vi "main.vi"() -> ()   [LabVIEW 2011]
doc: "Use this template to build a producer/consumer design pattern. Use this template when you need to execute a process, such as data analysis, when a data source, such as a triggered acquisition, produces data at an uneven rate and you need to execute the process when the data becomes available."
uses:
  <vilib>/httpClient/POSTBuffer.vi
  <vilib>/httpClient/LabVIEWHTTPClient.lvlib
  Labview-JSON/src/JSON.lvlib
  <vilib>/addons/internet/NI_InternetTK_FTP_VIs.lvlib
panel:
  in  "host":string
  in  "ftpPassword":string
  in  "ftpUsername":string
  out "# elements":i32=1
  out "Size queue flushed":i32=1
  out "Queue size [bytes]":i32=44
  in  "Queue size limit [Kbytes]":i32=10
  in  "url":string="localhost:3001/datas"
  in  "password":string
  in  "username":string
  in  "stop":bool
  out "data queue too large":T1={"acc1"=0.11785432029080489, "vel1"=0.881508362393591, "f1"=0.32413347839367, "timestamp"=3413457307.4501805, "system"="system01"}
  out "data queue":T1={"acc1"=0.11785432029080489, "vel1"=0.881508362393591, "f1"=0.32413347839367, "timestamp"=3413457307.4501805, "system"="system01"}
  # "HTTP Config"
  # "FTP Config"
  # "Queue"
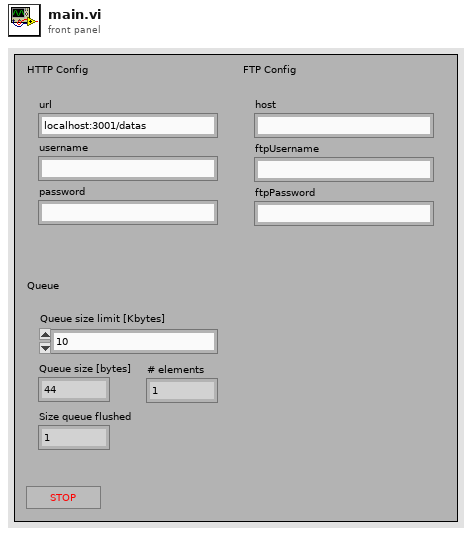
[diagram p1: front panel]
types:
  T1 = cluster{"acc1":dbl, "vel1":dbl, "f1":dbl, "timestamp":dbl, "system":string}
  T2 = cluster{"host":string, "ftpUsername":string, "ftpPassword":string, "ftpRemotePath":string}
  T3 = typedef "LabVIEWHTTPClient.lvlib/ClientHandle.ctl" = refnum<k1>
  T4 = enum16{"open", "replace", "create", "open or create", "replace or create", "replace or create with confirmation"}
  T5 = cluster{"acc1":dbl, "vel1":dbl, "f1":dbl, "timestamp":dbl, "system":string}[]
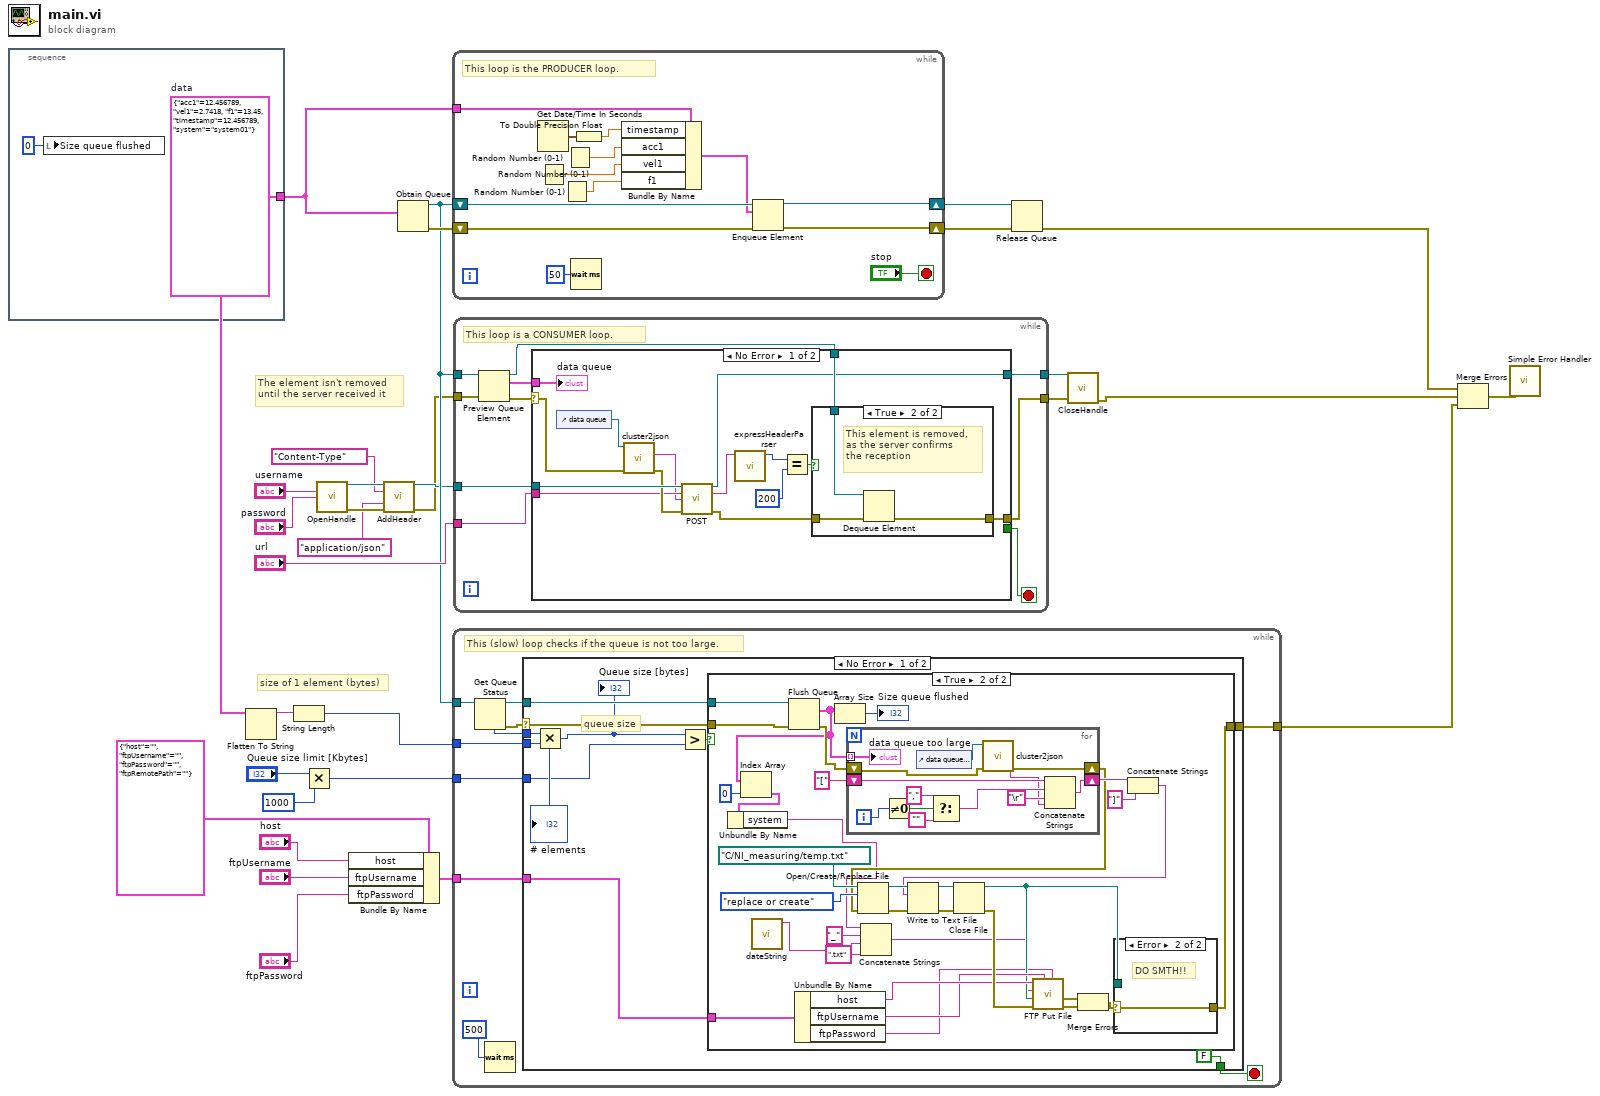
[diagram p0: block diagram]
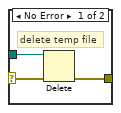
[diagram p3: hidden frame]
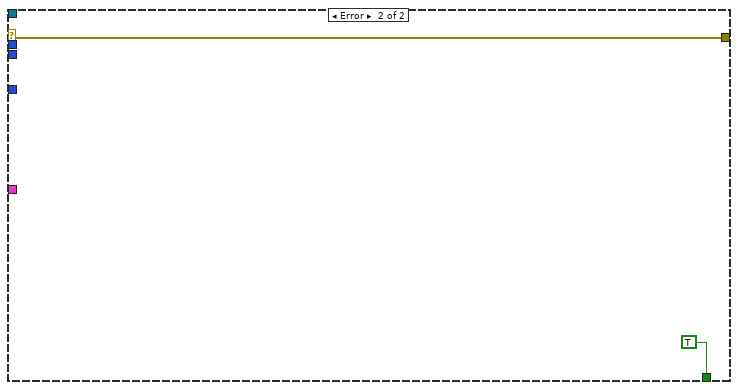
[diagram p4: hidden frame]
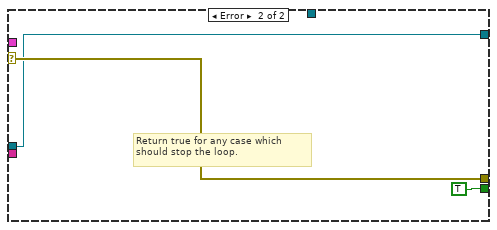
[diagram p6: hidden frame]
diagram:
  # "size of 1 element (bytes)"
  # "The element isn't removed \nuntil the server received it"
  n1 = stacked-sequence {
    tunnel: [w32] -> w21
    frame #0 {
      w32 = T1 {"acc1"=12.456789, "vel1"=2.7418, "f1"=13.45, "timestamp"=12.456789, "system"="system01"}  # data
      n2 = local write "Size queue flushed"(0 ("Size queue flushed")) -> ()
    }
  }
  n3 = Flatten To String(anything=w21) -> (data string=w20:string)  [unwired: 3 in, 2 out]
  n4 = String Length(string=w20) -> (length=w17:i32)
  n5 = Multiply(x="Queue size limit [Kbytes]", y=1000) -> (x*y=w16:i32)
  n6 = call <vilib>:"OpenHandle.vi"("username"="username", "password"="password") -> ("client handle out"=w6:T3, "error out"=w5:errorcluster)  [unwired: 12 in]
  n7 = Bundle By Name(cluster=T2 {"host"="", "ftpUsername"="", "ftpPassword"="", "ftpRemotePath"=""} ("input cluster"), "host"="host", "ftpUsername"="ftpUsername", "ftpPassword"="ftpPassword") -> (w7:T2)
  n8 = call <vilib>:"AddHeader.vi"("client handle"=w6, "header"="Content-Type", "value"="application/json", "error in (no error)"=w5) -> ("client handle out"=w4:T3, "error out"=w3:errorcluster)  [unwired: 10 in]
  n9 = Obtain Queue(element data type=w21) -> (queue out=w22:refnum<queue>, error out=w30:errorcluster)  [unwired: 4 in, 1 out]
  n10 = while {
    shift-right: [w41] -> w28
    shift-left: w30 -> [w42]
    shift-right: [w43] -> w29
    shift-left: w22 -> [w44]
    tunnel: w21 -> [w39]
    stop <- "stop" stop-if-true
    # "This loop is the PRODUCER loop."
    n11 = Get Date/Time In Seconds() -> (seconds since 1Jan1904=w38:timestamp)
    n12 = Random Number (0-1)() -> (number: 0 to 1=w34:dbl)
    n13 = Random Number (0-1)() -> (number: 0 to 1=w35:dbl)
    n14 = Random Number (0-1)() -> (number: 0 to 1=w36:dbl)
    n15 = Wait (ms)(milliseconds to wait=u32 50) -> ()  [unwired: 1 out]
    n16 = To Double Precision Float(number=w38) -> (double precision float=w37:dbl)
    n17 = Bundle By Name(cluster=w39, "timestamp"=w37, "acc1"=w36, "vel1"=w34, "f1"=w35) -> (w33:T1)
    n18 = Enqueue Element(queue=w44, element=w33, error in (no error)=w42) -> (queue out=w43:refnum<queue>, error out=w41:errorcluster)  [unwired: 1 in, 1 out]
  }
  n19 = while {
    tunnel: w22 -> [w55]
    tunnel: w17 -> [w52]
    tunnel: w16 -> [w51]
    tunnel: [w50] -> w15
    tunnel: w7 -> [w48]
    stop <- w46 stop-if-true
    # "This (slow) loop checks if the queue is not too large."
    n20 = Get Queue Status(queue=w55) -> (queue out=w54:refnum<queue>, error out=w47:errorcluster, # elements in queue=w53:i32)  [unwired: 2 in, 5 out]
    n21 = Wait (ms)(milliseconds to wait=u32 500) -> ()  [unwired: 1 out]
    n22 = case shown="No Error" w47 {
      selector: w47 -> [w57 w118]
      tunnel: w54 -> [w65 _]
      tunnel: w53 -> [w63 _]
      tunnel: w52 -> [w62 _]
      tunnel: w51 -> [w60 _]
      tunnel: [w59 w118] -> w50
      tunnel: w48 -> [w58 _]
      tunnel: [FALSE TRUE] -> w46
      frame No Error {
        # "queue size"
        n23 = Multiply(x=w63, y=w62) -> (x*y=w61:i32)
        "Queue size [bytes]" <- w61
        n24 = Greater?(x=w61, y=w60) -> (0:w64:bool)
        n25 = case shown="True" w64 {
          tunnel: w65 -> [_ w99]
          tunnel: w57 -> [w66 w98]
          tunnel: [w66 w95] -> w59
          tunnel: w58 -> [_ w94]
          frame False {
          }
          frame True {
            n26 = call "dateString.vi"() -> ("dateOUT"=w69:string)  [unwired: 11 in]
            n27 = Flush Queue(queue=w99, error in (no error)=w98) -> (remaining elements=w74:T5, error out=w78:errorcluster)  [unwired: 1 out]
            n28 = Index Array(array=w74, index=0) -> (element=w72:T1)
            n29 = Unbundle By Name(w72) -> ("system"=w71:string)
            n30 = Unbundle By Name(w94) -> ("host"=w93:string, "ftpUsername"=w92:string, "ftpPassword"=w75:string)
            n31 = Array Size(array=w74) -> (size(s)=→"Size queue flushed":i32)
            n32 = for {
              tunnel: w74 -> [w112] mode=indexing
              shift-right: [w104] -> w86
              shift-left: "[" -> [w106]
              shift-right: [w100] -> w77
              shift-left: w78 -> [w101]
              i -> [w107]
              n33 = Not Equal To 0?(x=w107) -> (x != 0?=w108:bool)
              n34 = control-ref of="data queue too large"() -> (w111:refnum<vi>)
              n35 = Select(t=",", s=w108, f="") -> (s? t:f=w105:string)
              n36 = call "cluster2json.vi"("error in"=w101, "Cluster Ref in"=w111) -> ("error out"=w100:errorcluster, "JSON"=w102:string)  [unwired: 7 in, 1 out]
              n37 = Concatenate Strings(w106, w105, "\r", w102) -> (w104:string)
              "data queue too large" <- w112
            }
            n38 = Open/Create/Replace File(file path (use dialog)=path "C:/NI_measuring/temp.txt", error in=w77, operation (0:open)=T4."replace or create") -> (refnum out=w82:refnum<file>, error out=w81:errorcluster)  [unwired: 3 in, 1 out]
            n39 = Concatenate Strings(w71, "_" ("string"), w69, ".txt" ("string")) -> (w67:string)
            n40 = Concatenate Strings(w86, "]") -> (w80:string)
            n41 = Write to Text File(file (use dialog)=w82, text=w80, error in=w81) -> (refnum out=w83:refnum<file>, error out=w84:errorcluster)  [unwired: 1 in, 1 out]
            n42 = Close File(refnum=w83, error in=w84) -> (path=w76:path, error out=w96:errorcluster)
            n43 = call <vilib>:"FTP Put File.vi"("password"=w75, "user"=w92, "error in (no error)"=w96, "local path"=w76, "remote path"=w67, "host"=w93) -> ("error out"=w91:errorcluster, "file error"=w90:errorcluster)  [unwired: 4 in]
            n44 = Merge Errors(w90, w91) -> (w89:errorcluster)
            n45 = case shown="Error" w89 {
              selector: w89 -> [w113 w116]
              tunnel: w76 -> [w114 _]
              tunnel: [w115 w116] -> w95
              frame No Error {
                # "delete temp file"
                n46 = Delete(path (use dialog)=w114, error in=w113) -> (error out=w115:errorcluster)  [unwired: 3 in, 2 out]
              }
              frame Error {
                # "DO SMTH!!"
              }
            }
          }
        }
        "# elements" <- w63
      }
      frame Error {
      }
    }
  }
  n47 = while {
    tunnel: w22 -> [w122]
    tunnel: w3 -> [w126]
    tunnel: w4 -> [w125]
    tunnel: "url" -> [w124]
    tunnel: [w123] -> w14
    tunnel: [w121] -> w12
    stop <- w120 stop-if-true
    # "This loop is a CONSUMER loop."
    n48 = Preview Queue Element(queue=w122, error in (no error)=w126) -> (queue out=w119:refnum<queue>, element=w127:T1, error out=w128:errorcluster)  [unwired: 1 in, 1 out]
    n49 = case shown="No Error" w128 {
      selector: w128 -> [w142 w149]
      tunnel: w127 -> [w135 _]
      tunnel: [_ TRUE] -> w120
      tunnel: w125 -> [w143 w148]
      tunnel: w124 -> [w140 _]
      tunnel: [w139 w149] -> w123
      tunnel: w119 -> [w137 _]
      tunnel: [w136 w148] -> w121
      frame No Error {
        n50 = control-ref of="data queue"() -> (w134:refnum<vi>)
        n51 = call "cluster2json.vi"("error in"=w142, "Cluster Ref in"=w134) -> ("error out"=w141:errorcluster, "JSON"=w129:string)  [unwired: 7 in, 1 out]
        n52 = call-poly <vilib>:"POST.vi"("client handle"=w143, "url"=w140, "data"=w129, "error in (no error)"=w141) -> ("client handle out"=w136:T3, "headers"=w132:string, "error out"=w138:errorcluster)  [unwired: 8 in, 1 out]
        n53 = call "expressHeaderParser.vi"("Header"=w132) -> ("Status code"=w131:i32)  [unwired: 10 in]
        n54 = Equal?(x=w131, y=200) -> (x = y?=w133:bool)
        n55 = case shown="True" w133 {
          tunnel: [w144 w147] -> w139
          tunnel: w138 -> [w144 w146]
          tunnel: w137 -> [_ w145]
          frame False {
          }
          frame True {
            # "This element is removed, \nas the server confirms \nthe reception"
            n56 = Dequeue Element(queue=w145, error in (no error)=w146) -> (error out=w147:errorcluster)  [unwired: 1 in, 3 out]
          }
        }
        "data queue" <- w135
      }
      frame Error {
        # "Return true for any case which should stop the loop."
      }
    }
  }
  n57 = Release Queue(queue=w29, error in (no error)=w28) -> (error out=w24:errorcluster)  [unwired: 1 in, 2 out]
  n58 = call <vilib>:"CloseHandle.vi"("client handle"=w12, "error in (no error)"=w14) -> ("error out"=w13:errorcluster)  [unwired: 13 in]
  n59 = Merge Errors(w24, w13, w15) -> (w23:errorcluster)
  n60 = call <vilib>:"Simple Error Handler.vi"("error in (no error)"=w23) -> ()  [unwired: 4 in, 5 out]
